vi "InitHandler.vi"(8 "Error Input":errorcluster) -> (0 "Error Output":errorcluster, 1 "Queue Out":refnum<queue>, 3 "AgentMessageEventHandler":refnum<k24>)   [LabVIEW 2017, in "LiteAgentSDK.lvlib"]
uses:
  LiteAgentSDK.lvlib
  C:/Users/Jan/Projects/LiteAgentSDK-LabVIEW/Source/Bin/LiteAgentSDK.LabVIEW.dll
  Bin/LiteAgentSDK.LabVIEW.dll
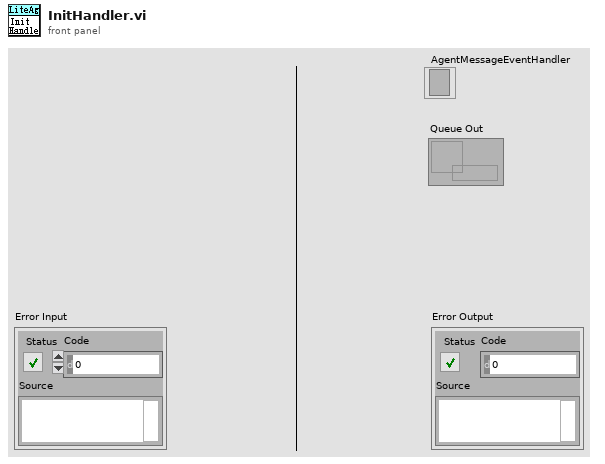
[diagram p1: front panel]
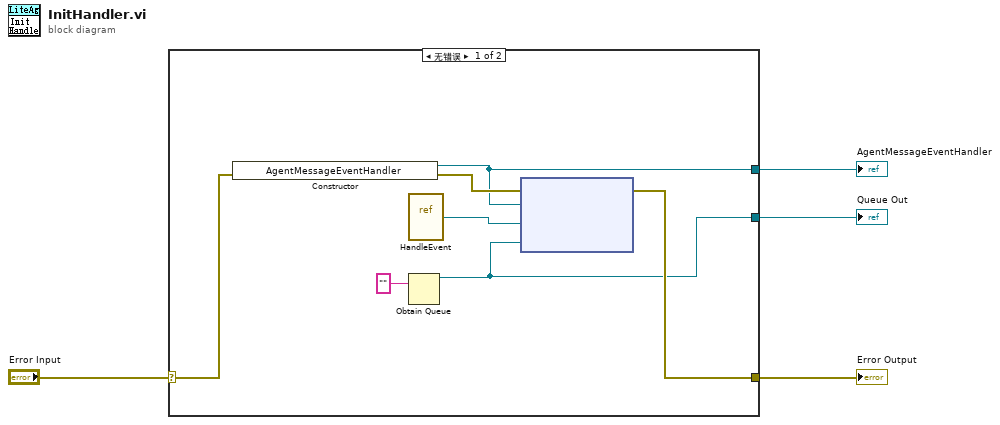
[diagram p0: block diagram]
diagram:
  n1 = case shown="无错误" "Error Input" {
    selector: "Error Input" -> [w11 w12]
    tunnel: [w7 w12] -> w3
    tunnel: [w8 _] -> w2
    tunnel: [w5 _] -> w1
    frame No Error {
      n2 = constructor class="AgentMessageEventHandler"(error in=w11) -> (reference out=w8:refnum<k24>, error out=w9:errorcluster)  [unwired: 2 in, 1 out]
      n3 = vi-ref "HandleEvent.vi"() -> ("vi reference"=w10:refnum<vi>)
      n4 = Obtain Queue(element data type="") -> (queue out=w5:refnum<queue>)  [unwired: 4 in, 2 out]
      n5 = node(w9, w8, w10, w5) -> (w7:errorcluster)  [unwired: 1 in, 1 out]
    }
    frame Error {
    }
  }
  "Error Output" <- w3
  "AgentMessageEventHandler" <- w2
  "Queue Out" <- w1
